vi "UpdateCVT[Acquire].vi"(8 "error in (no error)":errorcluster, 11 "Photometrics_CH-250_Cam in":refnum<class "Photometrics_CH-250_Cam.lvclass">) -> (0 "error out":errorcluster, 3 "Photometrics_CH-250_Cam in 2":refnum<class "Photometrics_CH-250_Cam.lvclass">)   [LabVIEW 2013, in "Photometrics_CH-250_Cam.lvclass"]
uses:
  Photometrics_CH-250_Cam.lvclass
  shared/Cameras/GenericCameraClass/GenericCamera.lvclass
  Photometrics_CH-250_Cam.lvclass/Photometrics_CH-250_Cam.ctl
  shared/CompressAndUpdate(Poly)/CompressAndUpdate(Numeric).vi
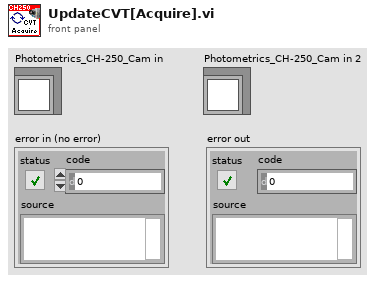
[diagram p1: front panel]
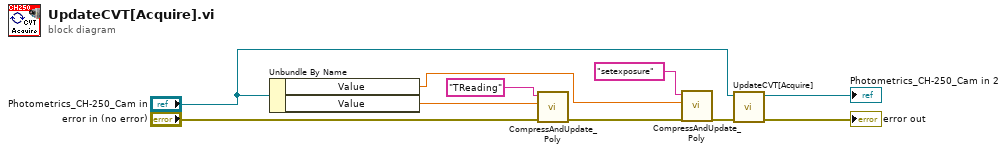
[diagram p0: block diagram]
diagram:
  n1 = Unbundle By Name("Photometrics_CH-250_Cam in") -> ("Value"=w1:dbl, "Value"=w10:dbl)
  n2 = call-poly "CompressAndUpdate_Poly.vi"("error in"="error in (no error)", "Numeric"=w10, "command or variable name"="TReading") -> ("error out"=w4:errorcluster)  [unwired: 8 in]
  n3 = call-poly "CompressAndUpdate_Poly.vi"("error in"=w4, "Numeric"=w1, "command or variable name"="setexposure") -> ("error out"=w3:errorcluster)  [unwired: 8 in]
  n4 = call-parent "UpdateCVT[Acquire].vi"("error in (no error)"=w3, "GenericCamera in"="Photometrics_CH-250_Cam in") -> ("error out"=→"error out":errorcluster, "GenericCamera out"=→"Photometrics_CH-250_Cam in 2":refnum<class "Photometrics_CH-250_Cam.lvclass">)  [unwired: 8 in]
